vi "L--end Sw.vi"(6 "Command Info In":T2, 8 "L--end Sw":T1={"1d"=48.0, "1s"=0.8, "2t"=3.0, "3a"=90.0, "4d"=0.0, "4s"=0.0}, 9 "Switch":string) -> (0 "Command Info Out":T2)   [LabVIEW 2017]
uses:
  <vilib>/Rock Robotics/WPI/Framework/Command Status Info.ctl
  <vilib>/Rock Robotics/WPI/Framework/Completion Status.ctl
  <vilib>/Rock Robotics/WPI/Framework/Completion Notifier.ctl
  Block Clusters/L--end Sw.ctl
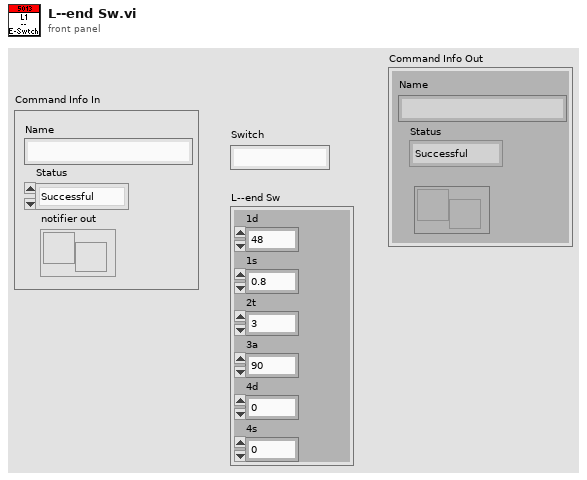
[diagram p1: front panel]
types:
  T1 = typedef "L--end Sw.ctl" = cluster{"1d":dbl, "1s":dbl, "2t":dbl, "3a":dbl, "4d":dbl, "4s":dbl}
  T2 = typedef "Command Status Info.ctl" = cluster{"Name":string, "Status":T3, "notifier out":T4}
  T3 = typedef "Completion Status.ctl" = enum16{"Successful", "Aborted", "Incomplete"}
  T4 = typedef "Completion Notifier.ctl" = refnum<notifier>
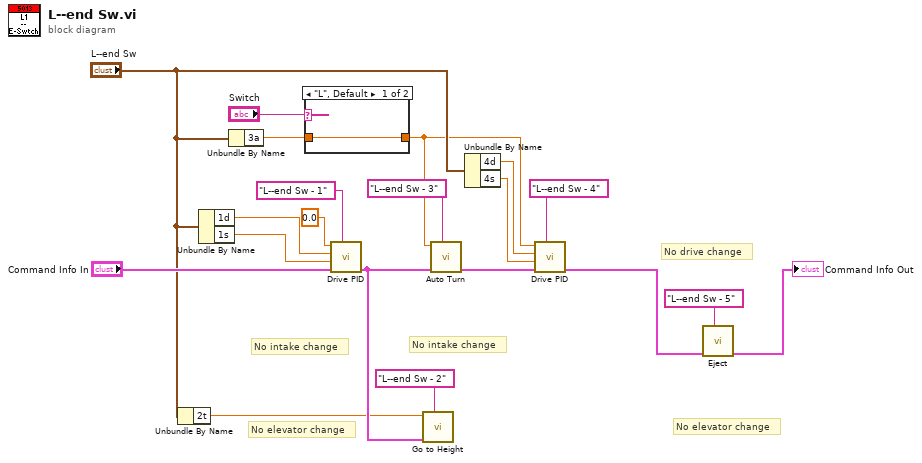
[diagram p0: block diagram]
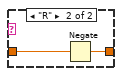
[diagram p2: hidden frame]
diagram:
  # "No drive change"
  # "No elevator change"
  # "No intake change"
  # "No intake change"
  # "No elevator change"
  n1 = Unbundle By Name("L--end Sw") -> ("2t"=w14:dbl)
  n2 = Unbundle By Name("L--end Sw") -> ("1d"=w16:dbl, "1s"=w15:dbl)
  n3 = Unbundle By Name("L--end Sw") -> ("3a"=w19:dbl)
  n4 = case shown="\"L\", Default" "Switch" {
    tunnel: [w21 w23] -> w3
    tunnel: w19 -> [w21 w22]
    frame "L", Default {
    }
    frame "R" {
      n5 = Negate(x=w22) -> (-x=w23:dbl)
    }
  }
  n6 = call "Drive PID.vi"("Description"="L--end Sw - 1", "Command Info In"="Command Info In", "Speed"=w15, "Distance"=w16, "Target Angle"=0.0 ("Distance")) -> ("Command Info Out"=w20:T2)  [unwired: 6 in]
  n7 = call "Go to Height.vi"("Description"="L--end Sw - 2", "Command Info In"=w20, "Target Height (in)"=w14) -> ()  [unwired: 8 in, 1 out]
  n8 = call "Auto Turn.vi"("Description"="L--end Sw - 3", "Command Info In"=w20, "Target Angle"=w3) -> ("Command Info Out"=w7:T2)  [unwired: 8 in]
  n9 = Unbundle By Name("L--end Sw") -> ("4d"=w2:dbl, "4s"=w1:dbl)
  n10 = call "Drive PID.vi"("Description"="L--end Sw - 4", "Command Info In"=w7, "Speed"=w1, "Distance"=w2, "Target Angle"=w3) -> ("Command Info Out"=w6:T2)  [unwired: 6 in]
  n11 = call "Eject.vi"("Description"="L--end Sw - 5", "Command Info In"=w6) -> ("Command Info Out"=→"Command Info Out":T2)  [unwired: 9 in]
